vi "Read Values cluster.vi"(8 "error in (no error)":errorcluster, 11 "WeatherSensor in":refnum<class "WeatherSensor.lvclass">) -> (0 "error out":errorcluster, 2 "Values cluster":T1, 3 "WeatherSensor out":refnum<class "WeatherSensor.lvclass">)   [LabVIEW 2018, in "WeatherSensor.lvclass"]
uses:
  WeatherSensor.lvclass
  WeatherSensor.lvclass/WeatherSensor.ctl
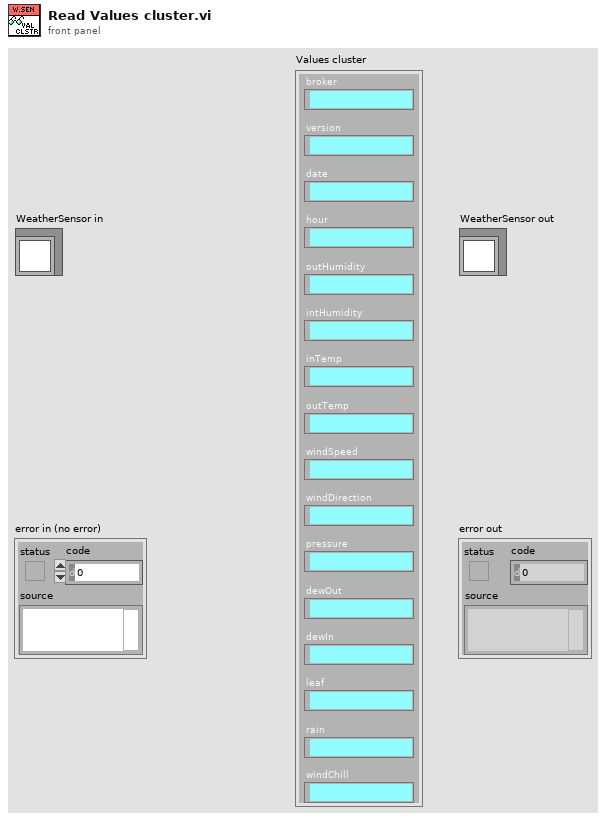
[diagram p1: front panel]
types:
  T1 = cluster{"broker":string, "version":string, "date":string, "hour":string, "outHumidity":string, "intHumidity":string, "inTemp":string, "outTemp":string, "windSpeed":string, "windDirection":string, "pressure":string, "dewOut":string, "dewIn":string, "leaf":string, "rain":string, "windChill":string}
  T2 = cluster{"broker":string, "version":string, "date":string, "hour":string, "outHumidity":string, "inHumidity":string, "inTemp":string, "outTemp":string, "windSpeed":string, "windDirection":string, "pressure":string, "dewOut":string, "dewIn":string, "leaf":string, "rain":string, "windChill":string}
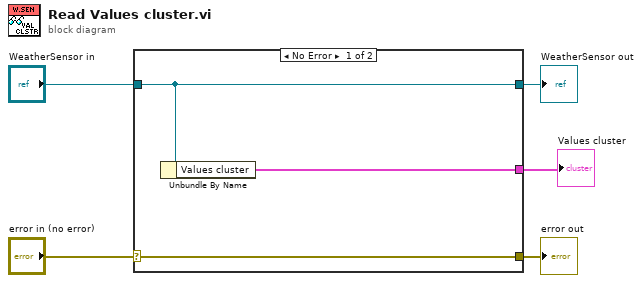
[diagram p0: block diagram]
diagram:
  n1 = case shown="No Error" "error in (no error)" {
    selector: "error in (no error)" -> [w8 w9]
    tunnel: [w8 w9] -> w4
    tunnel: [w7 w10] -> w2
    tunnel: "WeatherSensor in" -> [w7 w10]
    tunnel: [w6 _] -> w1
    frame No Error {
      n2 = Unbundle By Name(w7) -> ("Values cluster"=w6:T2)
    }
    frame Error {
    }
  }
  "error out" <- w4
  "WeatherSensor out" <- w2
  "Values cluster" <- w1
